vi "BRig_Host__Loop_Producer__tcp_System__Data_v4.vi"(0 "input_strCmd":string, 1 "input_I_SentCmd":bool) -> ()   [LabVIEW 2014]
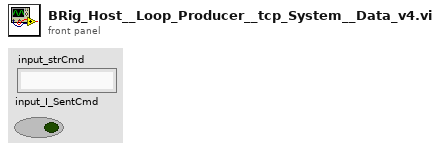
[diagram p1: front panel]
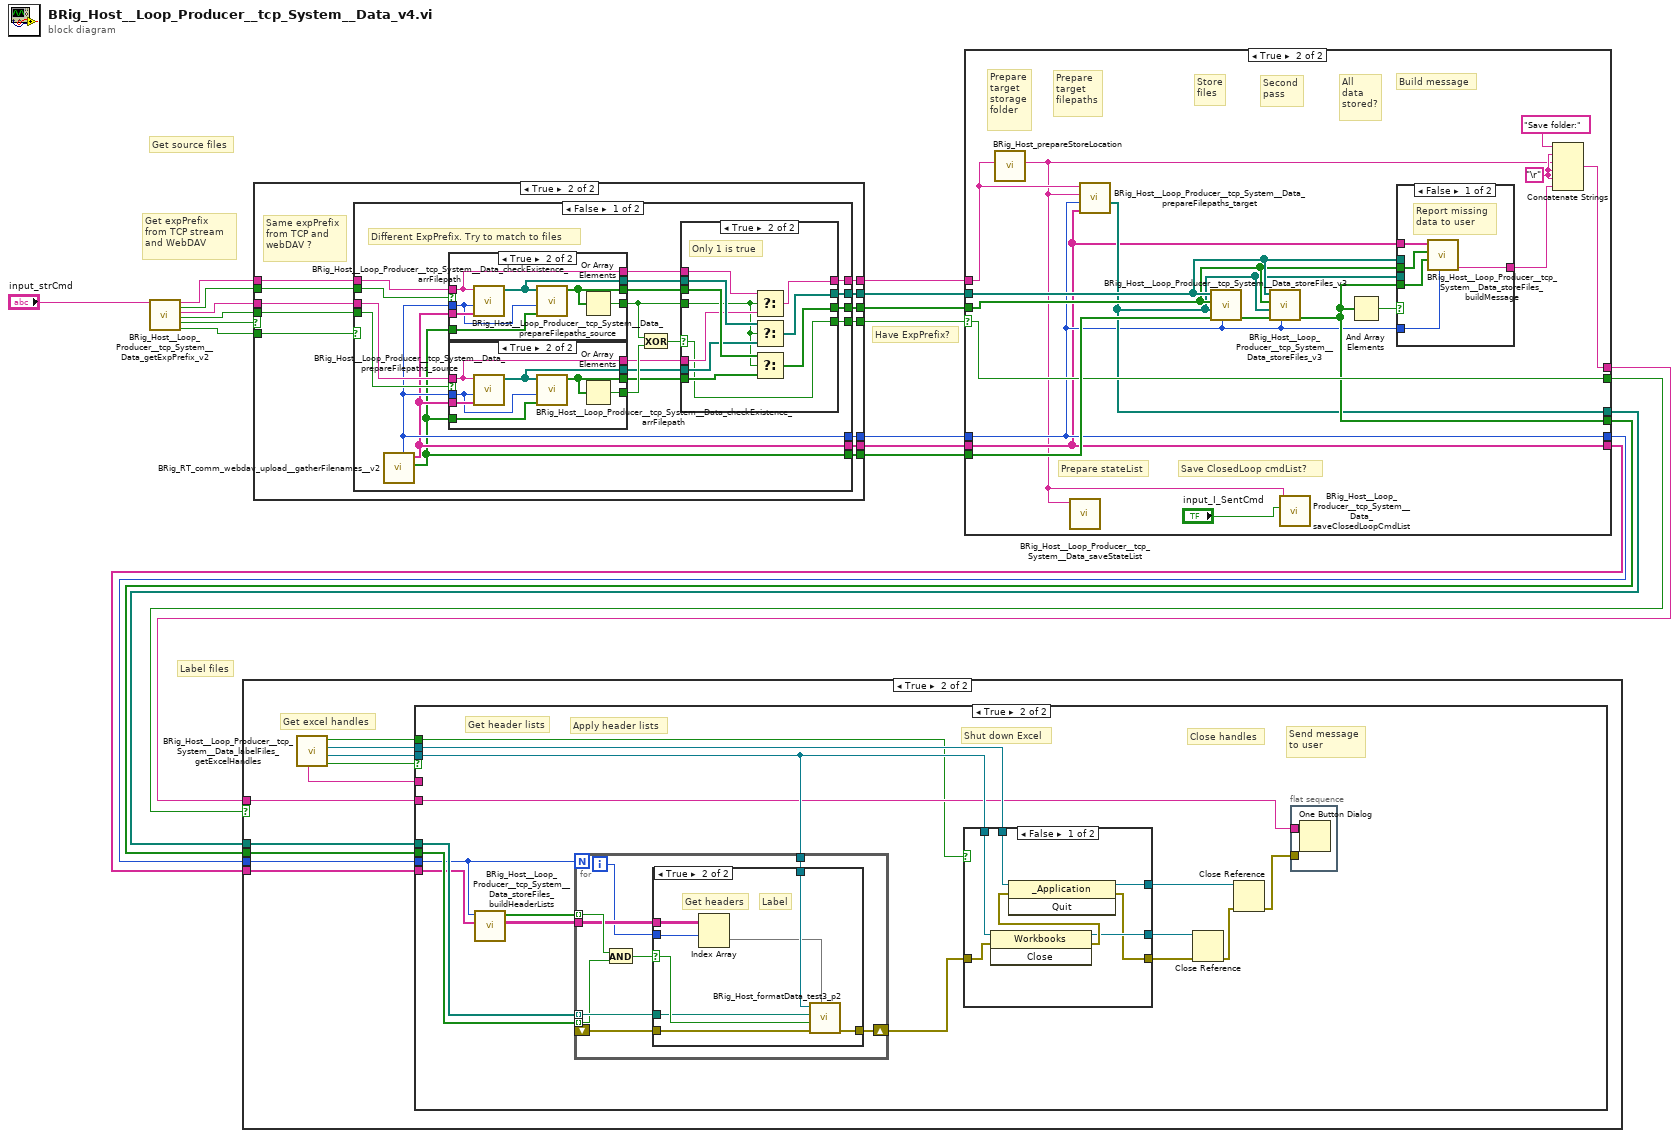
[diagram p0: block diagram]
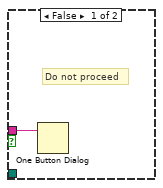
[diagram p2: hidden frame]
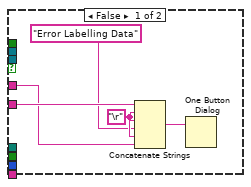
[diagram p3: hidden frame]
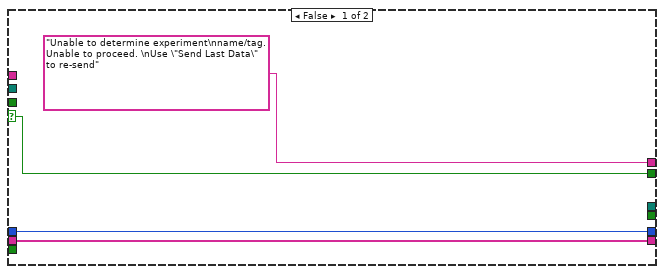
[diagram p6: hidden frame]
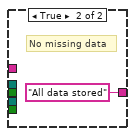
[diagram p7: hidden frame]
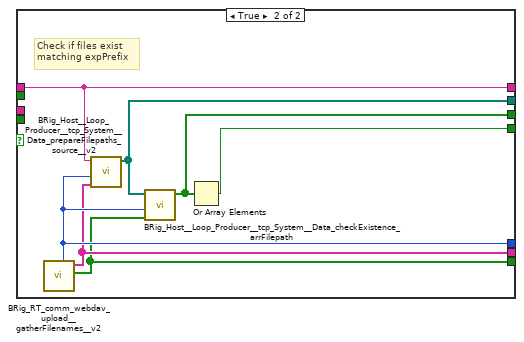
[diagram p12: hidden frame]
diagram:
  # "Label files"
  # "Have ExpPrefix?"
  # "Get expPrefix\nfrom TCP stream\nand WebDAV"
  # "Get source files"
  n1 = call "BRig_Host__Loop_Producer__tcp_System__Data_getExpPrefix_v2.vi"("input_strCmd"="input_strCmd") -> (14:"output_expPrefix_tcp"=w14:string, 15:"output_expPrefix_tcp"=w15:bool, 16:"output_expPrefix_webdav"=w16:string, 17:"output_expPrefix_webdav"=w17:bool, "output_expPrefix_any"=w19:bool, "output_expPrefix_same"=w18:bool)  [unwired: 13 in]
  n2 = case shown="True" w19 {
    tunnel: w18 -> [_ w32]
    tunnel: w17 -> [_ w28]
    tunnel: w16 -> [_ w30]
    tunnel: w15 -> [_ w29]
    tunnel: w14 -> [_ w31]
    tunnel: [_ w27] -> w12
    tunnel: [_ w26] -> w11
    tunnel: [_ w25] -> w10
    tunnel: [_ w24] -> w13
    tunnel: [_ w23] -> w9
    tunnel: [_ w22] -> w8
    tunnel: [_ w21] -> w7
    frame False {
    }
    frame True {
      # "Same expPrefix\nfrom TCP and\nwebDAV ?"
      n3 = case shown="False" w32 {
        tunnel: w31 -> [w51 w84]
        tunnel: w30 -> [w50 _]
        tunnel: w29 -> [w52 _]
        tunnel: w28 -> [w49 _]
        tunnel: [w39 w84] -> w27
        tunnel: [w38 w83] -> w26
        tunnel: [w37 w82] -> w25
        tunnel: [w36 w81] -> w24
        tunnel: [w35 w80] -> w23
        tunnel: [w34 w79] -> w22
        tunnel: [w33 w78] -> w21
        frame False {
          # "Different ExpPrefix. Try to match to files"
          n4 = call "BRig_RT_comm_webdav_upload__gatherFilenames__v2.vi"() -> ("output_arrBlank"=w33:bool[], "output_arrFilenames"=w34:string[], "output_n"=w35:i32)  [unwired: 9 in]
          n5 = case shown="True" w52 {
            tunnel: w51 -> [_ w74]
            tunnel: w35 -> [_ w76]
            tunnel: w34 -> [_ w77]
            tunnel: w33 -> [_ w75]
            tunnel: [_ w74] -> w46
            tunnel: [_ w73] -> w45
            tunnel: [_ w72] -> w44
            tunnel: [_ w71] -> w40
            frame False {
            }
            frame True {
              n6 = call "BRig_Host__Loop_Producer__tcp_System__Data_prepareFilepaths_source.vi"("input_arrFilenames"=w77, "input_nFilenames"=w76, "input_expPrefix"=w74) -> ("output_arrPath"=w73:path[])  [unwired: 8 in]
              n7 = call "BRig_Host__Loop_Producer__tcp_System__Data_checkExistence_arrFilepath.vi"("input_I_arrPath"=w75, "input_n"=w76, "input_arrPath"=w73) -> ("output_exist"=w72:bool[])  [unwired: 8 in]
              n8 = Or Array Elements(Boolean array=w72) -> (logical OR=w71:bool)
            }
          }
          n9 = case shown="True" w49 {
            tunnel: w50 -> [_ w67]
            tunnel: w35 -> [_ w69]
            tunnel: w34 -> [_ w70]
            tunnel: w33 -> [_ w68]
            tunnel: [_ w67] -> w43
            tunnel: [_ w66] -> w42
            tunnel: [_ w65] -> w41
            tunnel: [_ w64] -> w48
            frame False {
            }
            frame True {
              n10 = call "BRig_Host__Loop_Producer__tcp_System__Data_prepareFilepaths_source.vi"("input_arrFilenames"=w70, "input_nFilenames"=w69, "input_expPrefix"=w67) -> ("output_arrPath"=w66:path[])  [unwired: 8 in]
              n11 = call "BRig_Host__Loop_Producer__tcp_System__Data_checkExistence_arrFilepath.vi"("input_I_arrPath"=w68, "input_n"=w69, "input_arrPath"=w66) -> ("output_exist"=w65:bool[])  [unwired: 8 in]
              n12 = Or Array Elements(Boolean array=w65) -> (logical OR=w64:bool)
            }
          }
          n13 = Exclusive Or(1:w48, 2:w40) -> (0:w47:bool)
          n14 = case shown="True" w47 {
            selector: w47 -> [_ w53]
            tunnel: w46 -> [_ w63]
            tunnel: w45 -> [_ w62]
            tunnel: w44 -> [_ w61]
            tunnel: w43 -> [_ w60]
            tunnel: w42 -> [_ w59]
            tunnel: w41 -> [_ w58]
            tunnel: w40 -> [_ w57]
            tunnel: [_ w56] -> w39
            tunnel: [_ w55] -> w38
            tunnel: [_ w54] -> w37
            tunnel: [_ w53] -> w36
            frame False {
              # "Both false or both true\n\nIf false, can't proceed\nIf true, no way to choose"
            }
            frame True {
              # "Only 1 is true"
              n15 = Select(t=w63, s=w57, f=w60) -> (s? t:f=w56:string)
              n16 = Select(t=w62, s=w57, f=w59) -> (s? t:f=w55:path[])
              n17 = Select(t=w61, s=w57, f=w58) -> (s? t:f=w54:bool[])
            }
          }
        }
        frame True {
          # "Check if files exist\nmatching expPrefix"
          n18 = call "BRig_RT_comm_webdav_upload__gatherFilenames__v2.vi"() -> ("output_arrBlank"=w78:bool[], "output_arrFilenames"=w79:string[], "output_n"=w80:i32)  [unwired: 9 in]
          n19 = call "BRig_Host__Loop_Producer__tcp_System__Data_prepareFilepaths_source__v2.vi"("input_arrFilenames"=w79, "input_nFilenames"=w80, "input_expPrefix"=w84) -> ("output_arrPath"=w83:path[])  [unwired: 8 in]
          n20 = call "BRig_Host__Loop_Producer__tcp_System__Data_checkExistence_arrFilepath.vi"("input_I_arrPath"=w78, "input_n"=w80, "input_arrPath"=w83) -> ("output_exist"=w82:bool[])  [unwired: 8 in]
          n21 = Or Array Elements(Boolean array=w82) -> (logical OR=w81:bool)
        }
      }
    }
  }
  n22 = case shown="True" w13 {
    selector: w13 -> [w87 w95]
    tunnel: w12 -> [_ w105]
    tunnel: w11 -> [_ w101]
    tunnel: w10 -> [_ w100]
    tunnel: w9 -> [w85 w92]
    tunnel: w8 -> [w86 w91]
    tunnel: w7 -> [_ w104]
    tunnel: ["Unable to determine experiment\nname/tag. Unable to proceed. \nUse \"Send Last Data\" to re-send" ("message") w96] -> w3
    tunnel: [w87 w95] -> w4
    tunnel: [_ w94] -> w6
    tunnel: [_ w93] -> w5
    tunnel: [w85 w92] -> w2
    tunnel: [w86 w91] -> w1
    frame False {
    }
    frame True {
      w99 = "\r"
      # "Save ClosedLoop cmdList?"
      # "Build message"
      # "All\ndata\nstored?"
      # "Second\npass"
      # "Store\nfiles"
      # "Prepare stateList"
      # "Prepare\ntarget\nstorage\nfolder"
      # "Prepare\ntarget\nfilepaths"
      n23 = call "BRig_Host_prepareStoreLocation.vi"("input_expPrefix"=w105) -> ("output_folderPath"=w90:string)  [unwired: 9 in, 1 out]
      n24 = call "BRig_Host__Loop_Producer__tcp_System__Data_saveStateList.vi"("input_filepath_storage"=w90) -> ()  [unwired: 11 in]
      n25 = call "BRig_Host__Loop_Producer__tcp_System__Data_prepareFilepaths_target.vi"("input_arrFilenames"=w91, "input_nFilenames"=w92, "input_storagePath"=w90, "input_expPrefix"=w105) -> ("output_arrPath_target"=w93:path[])  [unwired: 7 in]
      n26 = call "BRig_Host__Loop_Producer__tcp_System__Data_storeFiles_v3.vi"("input_n"=w92, "input_stored"=w104, "input_arrPath_target"=w93, "input_exist_source"=w100, "input_arrPath_source"=w101) -> ("output_stored"=w103:bool[])  [unwired: 6 in]
      n27 = call "BRig_Host__Loop_Producer__tcp_System__Data_storeFiles_v3.vi"("input_n"=w92, "input_stored"=w103, "input_arrPath_target"=w93, "input_exist_source"=w100, "input_arrPath_source"=w101) -> ("output_stored"=w94:bool[])  [unwired: 6 in]
      n28 = call "BRig_Host__Loop_Producer__tcp_System__Data_saveClosedLoopCmdList.vi"("input_I_SentCmd"="input_I_SentCmd", "input_filepath_storage"=w90) -> ()  [unwired: 10 in]
      n29 = And Array Elements(Boolean array=w94) -> (logical AND=w102:bool)
      n30 = case shown="False" w102 {
        tunnel: w101 -> [_ _]
        tunnel: w100 -> [w109 _]
        tunnel: w93 -> [_ _]
        tunnel: w94 -> [w108 _]
        tunnel: w91 -> [w110 _]
        tunnel: w92 -> [w107 _]
        tunnel: [w106 "All data stored" ("output_msg")] -> w97
        frame False {
          # "Report missing\ndata to user"
          n31 = call "BRig_Host__Loop_Producer__tcp_System__Data_storeFiles_buildMessage.vi"("input_n"=w107, "input_stored"=w108, "input_exist_source"=w109, "input_arrFilenames"=w110) -> ("output_msg"=w106:string)  [unwired: 7 in]
        }
        frame True {
          # "No missing data"
        }
      }
      n32 = Concatenate Strings("Save folder:" ("string"), w99, w90, w99, w99, w97) -> (w96:string)
    }
  }
  n33 = case shown="True" w4 {
    tunnel: w6 -> [_ w115]
    tunnel: w5 -> [_ w114]
    tunnel: w3 -> [w112 w113]
    tunnel: w2 -> [_ w117]
    tunnel: w1 -> [_ w116]
    frame False {
      # "Do not proceed"
      n34 = One Button Dialog(message=w112) -> ()  [unwired: 1 in, 1 out]
    }
    frame True {
      # "Get excel handles"
      n35 = call "BRig_Host__Loop_Producer__tcp_System__Data_labelFiles_getExcelHandles.vi"() -> ("output_hExcel"=w122:bool, "output_hExcel_Workbooks"=w121:refnum<k7>, "output_hExcel_Application"=w120:refnum<k7>, "output_excel_runningPreviously"=w119:bool, "output_haveErrorMsg"=w118:string)  [unwired: 7 in]
      n36 = case shown="True" w122 {
        tunnel: w121 -> [_ w140]
        tunnel: w120 -> [_ w139]
        tunnel: w119 -> [_ w128]
        tunnel: w118 -> [w124 _]
        tunnel: w117 -> [_ w131]
        tunnel: w116 -> [_ w132]
        tunnel: w115 -> [_ w143]
        tunnel: w114 -> [_ w142]
        tunnel: w113 -> [w127 w133]
        frame False {
          w125 = "\r"
          n37 = Concatenate Strings(w127, w125, w125, "Error Labelling Data" ("string"), w125, w124) -> (w126:string)
          n38 = One Button Dialog(message=w126) -> ()  [unwired: 1 in, 1 out]
        }
        frame True {
          # "Send message\nto user"
          # "Close handles"
          # "Shut down Excel"
          # "Apply header lists"
          # "Get header lists"
          n39 = call "BRig_Host__Loop_Producer__tcp_System__Data_storeFiles_buildHeaderLists.vi"("input_arrFilenames"=w132, "input_nFilenames"=w131) -> (2:"output_HeaderLists"=w129:string[][], 3:"output_HeaderLists"=w130:bool[])  [unwired: 8 in]
          n40 = for {
            N: w131 -> [_]
            tunnel: w140 -> [w163]
            shift-right: [w162] -> w141
            shift-left: _ -> [w161]
            tunnel: w143 -> [w158] mode=indexing
            tunnel: w142 -> [w160] mode=indexing
            tunnel: w130 -> [w159] mode=indexing
            tunnel: w129 -> [w156]
            i -> [w155]
            n41 = And(x=w159, y=w158) -> (x .and. y?=w157:bool)
            n42 = case shown="True" w157 {
              selector: w157 -> [_ w169]
              tunnel: w163 -> [_ w172]
              tunnel: [w164 w171] -> w162
              tunnel: w161 -> [w164 w170]
              tunnel: w160 -> [_ w168]
              tunnel: w156 -> [_ w167]
              tunnel: w155 -> [_ w166]
              frame False {
              }
              frame True {
                # "Label"
                # "Get headers"
                n43 = Index Array(array=w167, index (row)=w166) -> (element=w165:string[])  [unwired: 1 in]
                n44 = call "BRig_Host_formatData_test3_p2.vi"("input_headers"=w165, "input_error"=w170, "input_Iexist"=w169, "input_filePath"=w168, "input_hdl_Workbooks"=w172) -> ("output_error"=w171:errorcluster)  [unwired: 4 in, 2 out]
              }
            }
          }
          n45 = case shown="False" w128 {
            tunnel: w141 -> [w150 w151]
            tunnel: w140 -> [w149 w152]
            tunnel: w139 -> [w147 w153]
            tunnel: [w146 w152] -> w138
            tunnel: [w145 w151] -> w137
            tunnel: [w144 w153] -> w136
            frame False {
              n46 = invoke class="Workbooks" method="Close"(reference=w149, error in=w150) -> (reference out=w146:refnum<k7>, error out=w148:errorcluster)  [unwired: 1 in, 1 out]
              n47 = invoke class="_Application" method="Quit"(reference=w147, error in=w148) -> (reference out=w144:refnum<k7>, error out=w145:errorcluster)  [unwired: 1 in, 1 out]
            }
            frame True {
            }
          }
          n48 = Close Reference(reference=w138, error in (no error)=w137) -> (error out=w135:errorcluster)
          n49 = Close Reference(reference=w136, error in (no error)=w135) -> (error out=w134:errorcluster)
          n50 = flat-sequence {
            tunnel: w134 -> [_]
            tunnel: w133 -> [w154]
            frame #0 {
              n51 = One Button Dialog(message=w154) -> ()  [unwired: 1 in, 1 out]
            }
          }
        }
      }
    }
  }
